vi "Create MTS Object.vi"(10 "Position":u32, 11 "RF Common Tests in":refnum<class "RF Common Tests.lvclass">) -> (0 "error out":errorcluster, 3 "SC Manufacturing Test out":refnum<class "SC Manufacturing Test.lvclass">)   [LabVIEW 2015, in "RF Common Tests.lvclass"]
doc: "Creates an MTS class object based upon position. Will read the MTS COM setting from the loaded recipe file."
uses:
  RF Common Tests.lvclass
  Classes/Manufacturing Test/Class/SC Manufacturing Test.lvclass
  Classes/Test Recipe/Class/Test Recipe.lvclass
  <vilib>/Cree, Inc/Cree Test Framework/Classes/Base Objects/Base Class/Base Class/Base Class.lvclass
  Classes/Application/Class/Application.lvclass
  Test Class/Test Class.lvclass
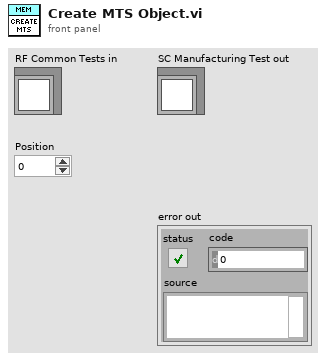
[diagram p1: front panel]
types:
  T1 = typedef "Application.lvlib/App Properties.lvclass/Class Properties -- Cluster.ctl" = cluster{"UUT Info":T2[], "Test Information":refnum<vi>, "Test Complete Event":refnum<user-event>, "Shop Floor System":refnum<class "Shop Floor System.lvclass">, "Gold Board":refnum<class "Golden Board.lvclass">, "Test Recipe":refnum<class "Test Recipe.lvclass">, "Instruments":refnum<class "Base Class.lvclass">[], "Mode":T3, "Test Results":cluster{"Pass":bool[], "Fail Codes":string[]}}
  T2 = typedef "Application.lvlib/App Properties.lvclass/UUT Reference -- Cluster.ctl" = cluster{"Serial Number Reference":refnum<vi>, "Status Message Reference":refnum<vi>}
  T3 = typedef "Application.lvlib/Application.lvclass/Op Mode -- Enum.ctl" = u16
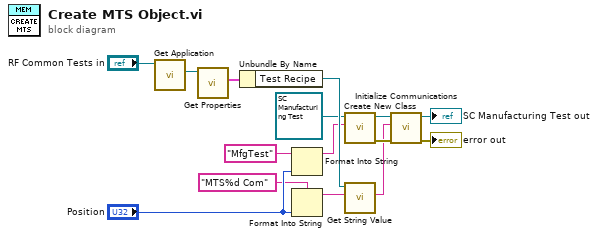
[diagram p0: block diagram]
diagram:
  n1 = call "Get Application.vi"("Test Class in"="RF Common Tests in") -> ("Application.lvlib:Application.lvclass"=w10:refnum<class "Application.lvclass">)  [unwired: 9 in, 1 out]
  n2 = call "Get Properties.vi"("Acrobat Template in"=w10) -> ("Class Properties"=w9:T1)  [unwired: 8 in, 2 out]
  n3 = Unbundle By Name(w9) -> ("Test Recipe"=w12:refnum<class "Test Recipe.lvclass">)
  n4 = Format Into String(initial string="MfgTest" ("Name"), "Position") -> (resulting string=w6:string)  [unwired: 2 in, 1 out]
  n5 = Format Into String(format string="MTS%d Com" ("Name"), "Position") -> (resulting string=w8:string)  [unwired: 2 in, 1 out]
  n6 = call <vilib>:"Create New Class.vi"("Name"=w6, "Base Class in"=refnum<class "SC Manufacturing Test.lvclass"> refnum ("SC Manufacturing Test.lvlib:SC Manufacturing Test.lvclass")) -> ("error out"=w3:errorcluster, "Base Class out"=w2:refnum<class "SC Manufacturing Test.lvclass">)  [unwired: 8 in]
  n7 = call "Get String Value.vi"("Name"=w8, "Test Recipe in"=w12) -> ("Value"=w1:string)  [unwired: 7 in, 2 out]
  n8 = call "Initialize Communications.vi"("error in (no error)"=w3, "COM Port"=w1, "Acrobat Template in"=w2) -> ("error out"=→"error out":errorcluster, "Acrobat Template out"=→"SC Manufacturing Test out":refnum<class "SC Manufacturing Test.lvclass">)  [unwired: 7 in]
